vi "processMsg.vi"(8 "error in (no error)":errorcluster, 10 "Pages":refnum<vi>[](array[refnum]), 11 "Msg in":string) -> (0 "error out":errorcluster, 3 "Msg out":string)   [LabVIEW 2017]
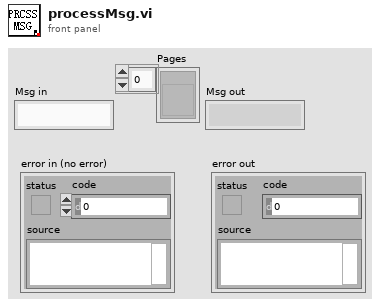
[diagram p1: front panel]
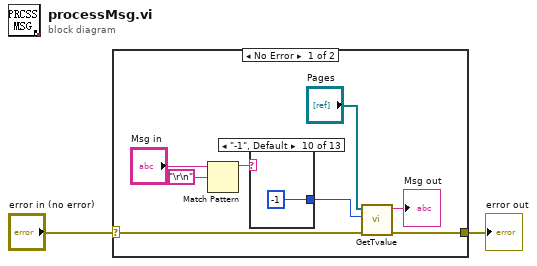
[diagram p0: block diagram]
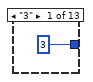
[diagram p2: hidden frame]
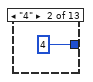
[diagram p3: hidden frame]
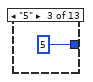
[diagram p4: hidden frame]
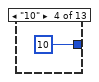
[diagram p5: hidden frame]
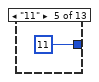
[diagram p6: hidden frame]
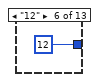
[diagram p7: hidden frame]
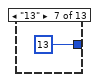
[diagram p8: hidden frame]
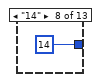
[diagram p9: hidden frame]
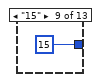
[diagram p10: hidden frame]
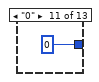
[diagram p11: hidden frame]
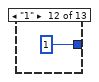
[diagram p12: hidden frame]
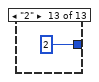
[diagram p13: hidden frame]
diagram:
  n1 = case shown="No Error" "error in (no error)" {
    selector: "error in (no error)" -> [w7 w24]
    tunnel: [w10 w24] -> w2
    frame No Error {
      n2 = Match Pattern(string="Msg in", regular expression="\r\n") -> (before substring=w4:string)  [unwired: 4 out]
      n3 = case shown="\"-1\", Default" w4 {
        tunnel: [3 4 5 10 11 12 13 14 15 -1 0 1 2] -> w9
        frame "3" {
        }
        frame "4" {
        }
        frame "5" {
        }
        frame "10" {
        }
        frame "11" {
        }
        frame "12" {
        }
        frame "13" {
        }
        frame "14" {
        }
        frame "15" {
        }
        frame "-1", Default {
        }
        frame "0" {
        }
        frame "1" {
        }
        frame "2" {
        }
      }
      n4 = call "GetTvalue.vi"("error in"=w7, "Numeric"=w9, "Pages"="Pages") -> ("error out"=w10:errorcluster, "T (K) or R"=→"Msg out":string)  [unwired: 5 out]
    }
    frame Error {
    }
  }
  "error out" <- w2
